vi "Close Device.vi"(8 "error in (no error)":errorcluster, 11 "ThorlabsLTS in":refnum<class "ThorlabsLTS.lvclass">) -> (0 "error out":errorcluster)   [LabVIEW 2020, in "ThorlabsLTS.lvclass"]
uses:
  ThorlabsLTS.lvclass
  ThorlabsLTS.lvclass/ThorlabsLTS.ctl
  C:/GEECS/Developers Version/builds/Device builds/ThorLabsLTS/Thorlabs.MotionControl.IntegratedStepperMotorsCLI.dll
  Thorlabs.MotionControl.IntegratedStepperMotorsCLI.dll
  C:/GEECS/Developers Version/builds/Device builds/ThorLabsLTS/Thorlabs.MotionControl.Controls.dll
  Thorlabs.MotionControl.Controls.dll
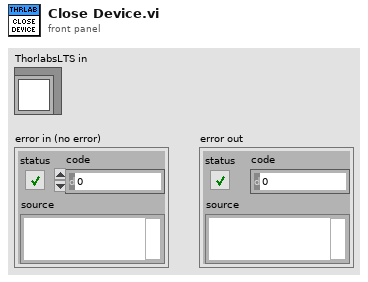
[diagram p1: front panel]
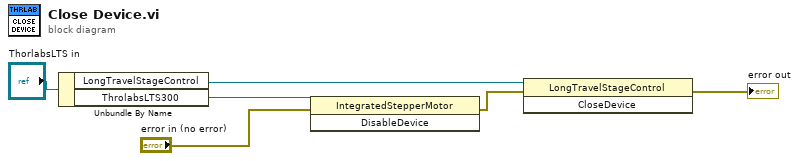
[diagram p0: block diagram]
diagram:
  n1 = Unbundle By Name("ThorlabsLTS in") -> ("LongTravelStageControl"=w4:refnum<k24>, "ThrolabsLTS300"=w3:refnum<k24>)
  n2 = invoke class="IntegratedStepperMotor" method="DisableDevice"(reference=w3, error in="error in (no error)") -> (error out=w1:errorcluster)  [unwired: 1 in, 2 out]
  n3 = invoke class="LongTravelStageControl" method="CloseDevice"(reference=w4, error in=w1) -> (error out=→"error out":errorcluster)  [unwired: 1 in, 2 out]
